vi "Post Substeps PWM Input Task.vi"(9 "Socket No":u16=1, 10 "PWM Input In":T1, 11 "Sequence Context In":refnum<k7>) -> (0 "error out":errorcluster, 1 "Duty Cycle":dbl[](array[numeric]), 2 "PWM Read":dbl[](array[numeric]), 3 "Report Text":string, 4 "Physical Channel":string[](array[string]))   [LabVIEW 2023, in "LTT_TeststandSteptypes.lvlib"]
doc: "This VI is Anaload Input Read MultiNumeric Test and PostSub Steptypes"
uses:
  LTT_TeststandSteptypes.lvlib
  HardwareAbstractionLayer_LVOOP/PWM Input/NI PWM Input_class/NI PWM DAQ/Control/PWMInputEdit.ctl
  HardwareAbstractionLayer_LVOOP/Main/Class Options.ctl
  HardwareAbstractionLayer_LVOOP/PWM Input/PWM Input_class/PWM Input.lvclass
  HardwareAbstractionLayer_LVOOP/Main/Main.lvclass
  HardwareAbstractionLayer_LVOOP/PWM Input/NI PWM Input_class/NI PWM Input.lvclass
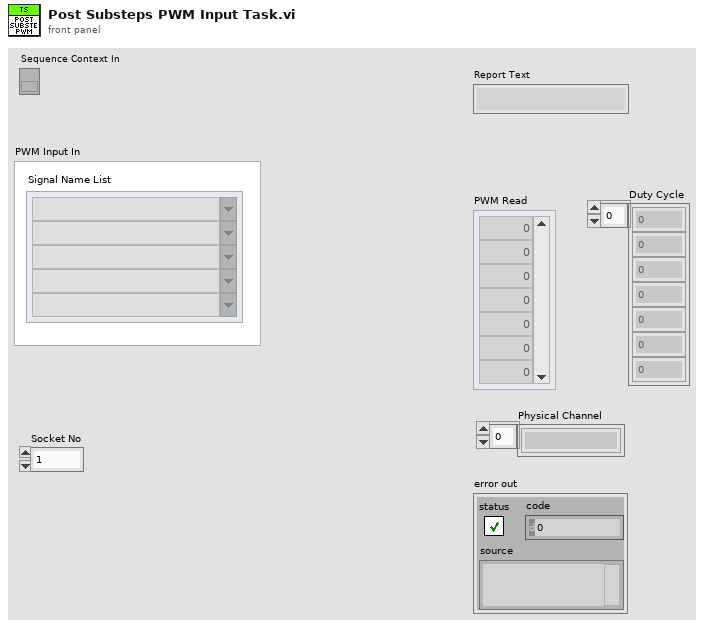
[diagram p1: front panel]
types:
  T1 = typedef "HardwareAbstractionLayer_LVOOP.lvlib/NI PWM Input.lvclass/PWMInputEdit.ctl" = cluster{"Signal Name List":string[]}
  T2 = typedef "HardwareAbstractionLayer_LVOOP.lvlib/Main.lvclass/Class Options.ctl" = enum16{"Init All Class", "Read All Class", "Write AI Class", "Write AO Class", "Write AO Waveform Generation", "Write DI Class", "Write DO Class", "Write PWM Input Class", "Write PWM Output Class", "Exit"}
  T3 = typedef "HardwareAbstractionLayer_LVOOP.lvlib/Main.lvclass/Class Ref.ctl" = cluster{"FGV":refnum<class "Function Global Variable.lvclass">, "Notifier":refnum<class "NotifierHandler.lvclass">, "Queue":refnum<class "Queue Handler.lvclass">, "User Event":refnum<class "User Event.lvclass">, "Data Manager":refnum<class "Data Manager.lvclass">, "DMM":refnum<class "DMM.lvclass">, "Function Generator":refnum<class "Function Generator.lvclass">, "Oscilloscope":refnum<class "Oscilloscope.lvclass">, "PowerSupply":refnum<class "PowerSupply.lvclass">, "Teststand":refnum<class "Teststand.lvclass">, "AO":refnum<class "AO.lvclass">, "AI":refnum<class "AI.lvclass">, "Database":refnum<class "Database.lvclass">, "AO Waveform Generation":refnum<class "AO.lvclass">, "DO":refnum<class "DO.lvclass">, "DI":refnum<class "DI.lvclass">, "PWM Output":refnum<class "PWM Output.lvclass">, "PWM Input":refnum<class "PWM Input.lvclass">, "RelayOutput":refnum<class "NISwitch.lvclass">, "Modbus":refnum<class "Modbus.lvclass">, "CAN":refnum<class "CAN.lvclass">}
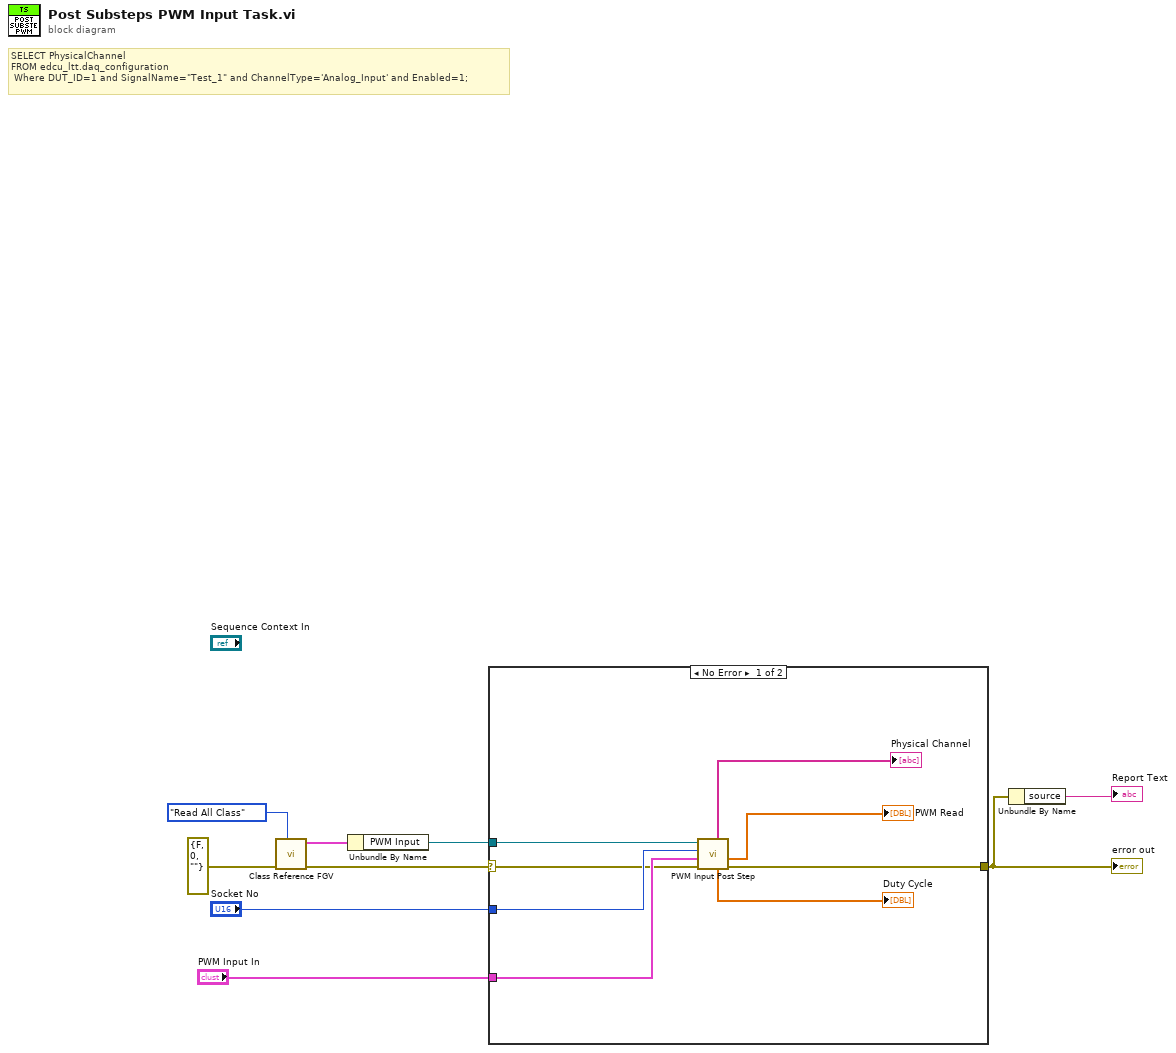
[diagram p0: block diagram]
diagram:
  # "SELECT PhysicalChannel \nFROM edcu_ltt.daq_configuration\n Where DUT_ID=1 and SignalName=\"Test_1\" and ChannelType='Analog_Input' and Enabled=1;"
  n1 = call "Class Reference FGV.vi"("Options"=Class_Options."Read All Class", "error in"=errorcluster {"status"=FALSE, "code"=0, "source"=""}) -> ("error out"=w6:errorcluster, "Class Cluster Out"=w8:T3)  [unwired: 8 in]
  n2 = Unbundle By Name(w8) -> ("PWM Input"=w1:refnum<class "PWM Input.lvclass">)
  n3 = case shown="No Error" w6 {
    selector: w6 -> [w12 w18]
    tunnel: w1 -> [w13 _]
    tunnel: [w17 w18] -> w2
    tunnel: "Socket No" -> [w15 _]
    tunnel: "PWM Input In" -> [w14 _]
    frame No Error {
      n4 = call-dynamic "PWM Input Post Step.vi"("error in (no error)"=w12, "PWM Input In"=w14, "Socket No"=w15, "PWM Input in"=w13) -> ("error out"=w17:errorcluster, "AnalogRead"=→"PWM Read":dbl[], "Duty Cycle"=→"Duty Cycle":dbl[], "Physical Channel"=→"Physical Channel":string[])  [unwired: 2 in, 2 out]
    }
    frame Error {
    }
  }
  "error out" <- w2
  n5 = Unbundle By Name(w2) -> ("source"=→"Report Text":string)
